vi "jModule - Initialize.vi"(4 "Wait on Module Timeout, ms (5000)":u32=5000, 6 "Wait on Module(s) (\"\": none)":string, 8 "error in (no error)":errorcluster, 9 "jMsgRxList":refnum<class "jMsg.lvclass">[](array[class]), 10 "jMsgTxList":refnum<class "jMsg.lvclass">[](array[class]), 11 "jModule Template_SubPanel UI (Right)":refnum<class "Module_SP_GameLeaderboard.lvclass">) -> (0 "error out":errorcluster, 3 "jModule Template_SubPanel UI (Right)":refnum<class "Module_SP_GameLeaderboard.lvclass">)   [LabVIEW 2019, in "Module_SP_GameLeaderboard.lvclass"]
doc: "This VI is used to intialize the jModule object. \n\nThis includes:\n* Creating the jRouter for the module (the queue for receiving the jMsgs)\n -- Max Queue Size intput limits the number of jMsgs that can back up\n* Adding this module to the subscription list of each message that this module expects to receive (<b>jMsgRxList</b> array)\n* Ensuring that the messages that this module will send (<b>jMsgTxList</b> array) have subscription lists created.\n* Initializing the Timeout for receiving messages to -1\n* Setting up the module to handle Batch jMsg sends\n* Adding the Module Name to the jModuleMasterTable\n* Waiting until every Module listed in the <b>Wait on Module(s)</b> has been added to the jModuleMasterTable\n* Sending out jMsg_Sys_JAMAModuleOnline\n\nNote that ALL modules are automatically registered to:\n* send JAMAException jMsgs\n* receive Shutdown jMsgsJSMA Module Template - SubPanels 0.2.0.9\nRob Humfeld - Jet Engineering\nCopyright (c) 2019, Jet Engineering"
uses:
  Module_SP_GameLeaderboard.lvclass
  C:/Program Files/National Instruments/LabVIEW 2019/user.lib/Jet Engineering/JSMA/Libraries/jModule Class/jModule.lvclass
  <userlib>/Jet Engineering/JSMA/Libraries/jMsg Class/jMsg.lvclass
  <userlib>/Jet Engineering/JSMA Signal Abstraction Layer (SAL)/CORE/jModule_SAL Class/jModule_SAL_ClientRxMsg STYP.ctl
  <userlib>/Jet Engineering/JSMA Signal Abstraction Layer (SAL)/CORE/jMsgs_CORE/jMsg_SAL_TagServiceDefinition/jMsg_SAL_TagServiceDefinition.lvclass
  <userlib>/Jet Engineering/JSMA Signal Abstraction Layer (SAL)/CORE/jMsgs_CORE/jMsg_SAL_TagDataPacket/jMsg_SAL_TagDataPacket.lvclass
  <userlib>/Jet Engineering/JSMA Signal Abstraction Layer (SAL)/CORE/jMsgs_CORE/jMsg_SAL_TagServiceAvailable/jMsg_SAL_TagServiceAvailable.lvclass
  <userlib>/Jet Engineering/JSMA Signal Abstraction Layer (SAL)/CORE/jModule_SAL Class/jModule_SAL_ClientTxMsg STYP.ctl
  <userlib>/Jet Engineering/JSMA Signal Abstraction Layer (SAL)/CORE/jMsgs_CORE/jMsg_SAL_TagServicePoll/jMsg_SAL_TagServicePoll.lvclass
  <userlib>/Jet Engineering/JSMA Signal Abstraction Layer (SAL)/CORE/jMsgs_CORE/jMsg_SAL_TagServiceRequest/jMsg_SAL_TagServiceRequest.lvclass
  <userlib>/Jet Engineering/JSMA/Libraries/jModule Class/jModule.lvclass/jModule.ctl
  <userlib>/Jet Engineering/JSMA/Libraries/jMsg Class/jMsg.lvclass/jMsg.ctl
  <userlib>/Jet Engineering/JSMA/Libraries/jSubscription Class/jSubscription.lvclass/jSubscription.ctl
  <userlib>/Jet Engineering/JSMA/Libraries/jRouter Class/jRouter.lvclass/jRouter.ctl
  <userlib>/Jet Engineering/JSMA/Libraries/jMsg_CORE/jMsg_JSMA_SubscriptionChange/jMsg_JSMA_SubscriptionChange.lvclass/jMsg_JSMA_SubscriptionChange.ctl
  <userlib>/Jet Engineering/JSMA/Libraries/jMsg Class/jMsg Get-Create Subscription List.vi
  <userlib>/Jet Engineering/JSMA/Libraries/jMsg Class/Read Name.vi
  <userlib>/Jet Engineering/JSMA/Libraries/jMasterTable_Message/jMasterTable_Message - Add jMsg.vi
  <userlib>/Jet Engineering/JSMA/Libraries/jMsg_CORE/jMsg_JSMA_SubscriptionChange/(create) jMsg_JSMA_SubscriptionChange.vi
  <userlib>/Jet Engineering/JSMA/Libraries/jModule Class/jModule - SimpleTx.vi
  <userlib>/Jet Engineering/JSMA/Libraries/jSubscription Class/(create) jSubscription.vi
  <userlib>/Jet Engineering/JSMA/Libraries/jSubscription_Background/(create) jSubscription_Background.vi
  <userlib>/Jet Engineering/JSMA/Libraries/jSubscription_Critical/(create) jSubscription_Critical.vi
  <userlib>/Jet Engineering/JSMA/Libraries/jMasterTable_Subscription/jMasterTable_Subscription - Add Subscription.vi
  <userlib>/Jet Engineering/JSMA/Libraries/jMasterTable_Subscription/jMasterTable_Subscription - Get-Create Queue.vi
  <userlib>/Jet Engineering/JSMA/Libraries/Shared/JSMA_GetClassName.vi
  <userlib>/Jet Engineering/JSMA/Libraries/jMasterTable_Message/jMasterTable_Message - Get-Create Queue.vi
  <userlib>/Jet Engineering/JSMA/Libraries/jMsg Class/(create) jMsg.vi
  <userlib>/Jet Engineering/JSMA/Libraries/jMasterTable_Subscription/jMasterTable_Subscription - Remove Module.vi
  <userlib>/Jet Engineering/JSMA/Libraries/jMsg Class/Write Source.vi
  <userlib>/Jet Engineering/JSMA/Libraries/jMasterTable_Subscription/jMasterTable_Subscription - Get Queue Type.vi
  <userlib>/Jet Engineering/JSMA/Libraries/jRouter Class/Read Module RxQueue.vi
  <userlib>/Jet Engineering/JSMA/Libraries/jSubscription Class/Get Module Name.vi
  <userlib>/Jet Engineering/JSMA/Libraries/jSubscription Class/Read jRouter.vi
  <userlib>/Jet Engineering/JSMA/Libraries/jRouter Class/Read Module Name.vi
  <userlib>/Jet Engineering/JSMA/Libraries/jMsg_CORE/jMsg_JSMA_SubscriptionChange/jMsg_JSMA_SubscriptionChange.lvclass
  C:/Program Files/National Instruments/LabVIEW 2019/user.lib/Jet Engineering/JSMA/Libraries/jMsg Class/jMsg.lvclass
  <vilib>/Utility/LVClass/Get LV Class Path.vi
  <userlib>/Jet Engineering/JSMA/Libraries/jModule Class/jModule - Prepare Addressed.vi
  <userlib>/Jet Engineering/JSMA/Libraries/jSubscription Class/jSubscription.lvclass
  <userlib>/Jet Engineering/JSMA/Libraries/jSubscription_Background/jSubscription_Background.lvclass
  <userlib>/Jet Engineering/JSMA/Libraries/jSubscription_Critical/jSubscription_Critical.lvclass
  <userlib>/Jet Engineering/JSMA GUISubPanel CORE/jModule_GUISubPanel.lvclass
  <userlib>/Jet Engineering/JSMA Signal Abstraction Layer (SAL)/CORE/jModule_SAL Class/jModule_SAL_ServerRxMsg STYP.ctl
  <userlib>/JET Engineering/JSMA Signal Abstraction Layer (SAL)/CORE/jModule_SAL Class/jModule_SAL.lvclass
  <userlib>/Jet Engineering/JSMA Signal Abstraction Layer (SAL)/CORE/jModule_SAL Class/jModule_SAL_ServerTxMsg STYP.ctl
  <userlib>/Jet Engineering/JSMA/Libraries/jModule Class/jModule.lvclass
  <userlib>/Jet Engineering/JSMA Signal Abstraction Layer (SAL)/CORE/jMsgs_CORE/jMsg_SAL_SignalUpdate/jMsg_SAL_SignalUpdate.lvclass
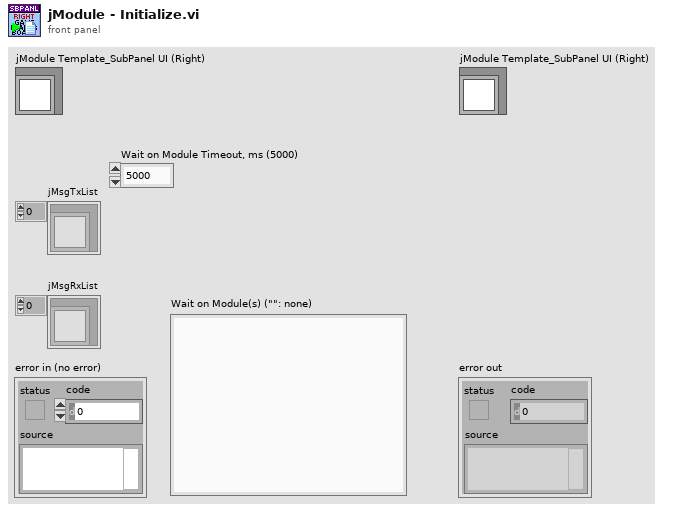
[diagram p1: front panel]
types:
  T1 = typedef "JSMA SAL CORE.lvlib/jModule_SAL.lvclass/jModule_SAL_ServerTxMsg STYP.ctl" = cluster{"jMsg_SAL_TagServiceDefinition":refnum<class "jMsg_SAL_TagServiceDefinition.lvclass">, "jMsg_SAL_TagDataPacket":refnum<class "jMsg_SAL_TagDataPacket.lvclass">, "jMsg_SAL_TagServiceAvailable":refnum<class "jMsg_SAL_TagServiceAvailable.lvclass">}
  T2 = typedef "JSMA SAL CORE.lvlib/jModule_SAL.lvclass/jModule_SAL_ServerRxMsg STYP.ctl" = cluster{"jMsg_SAL_TagServiceRequest":refnum<class "jMsg_SAL_TagServiceRequest.lvclass">, "jMsg_SAL_TagServicePoll":refnum<class "jMsg_SAL_TagServicePoll.lvclass">, "jMsg_SAL_SignalUpdate":refnum<class "jMsg_SAL_SignalUpdate.lvclass">}
  T3 = typedef "JSMA SAL CORE.lvlib/jModule_SAL.lvclass/jModule_SAL_ClientRxMsg STYP.ctl" = cluster{"jMsg_SAL_TagServiceDefinition":refnum<class "jMsg_SAL_TagServiceDefinition.lvclass">, "jMsg_SAL_TagDataPacket":refnum<class "jMsg_SAL_TagDataPacket.lvclass">, "jMsg_SAL_TagServiceAvailable":refnum<class "jMsg_SAL_TagServiceAvailable.lvclass">}
  T4 = typedef "JSMA SAL CORE.lvlib/jModule_SAL.lvclass/jModule_SAL_ClientTxMsg STYP.ctl" = cluster{"jMsg_SAL_TagServicePoll":refnum<class "jMsg_SAL_TagServicePoll.lvclass">, "jMsg_SAL_TagServiceRequest":refnum<class "jMsg_SAL_TagServiceRequest.lvclass">}
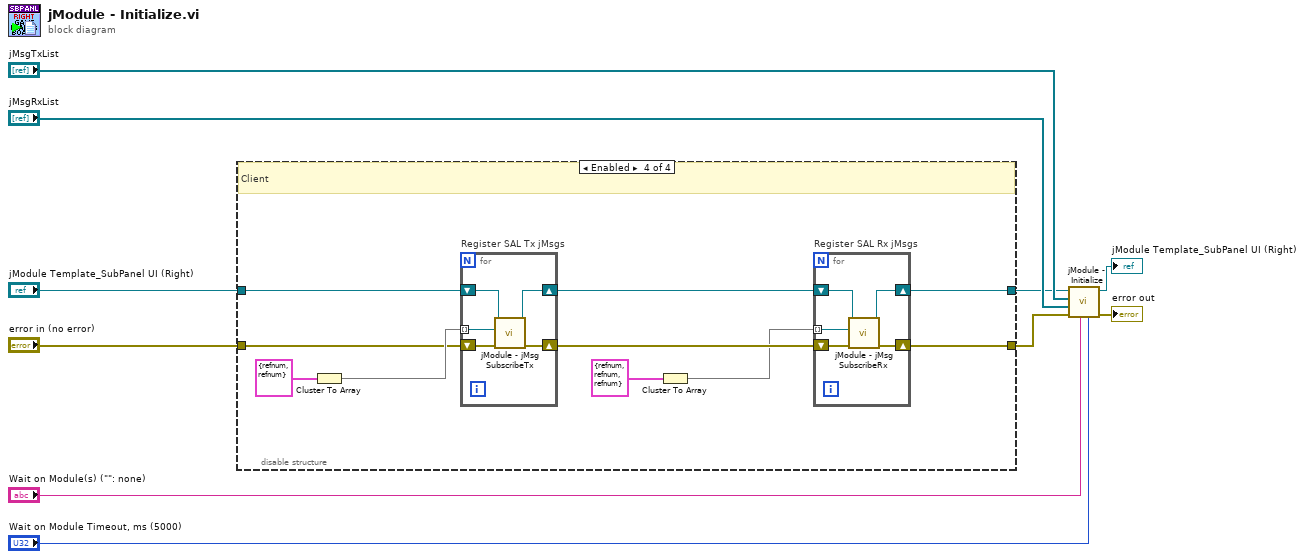
[diagram p0: block diagram]
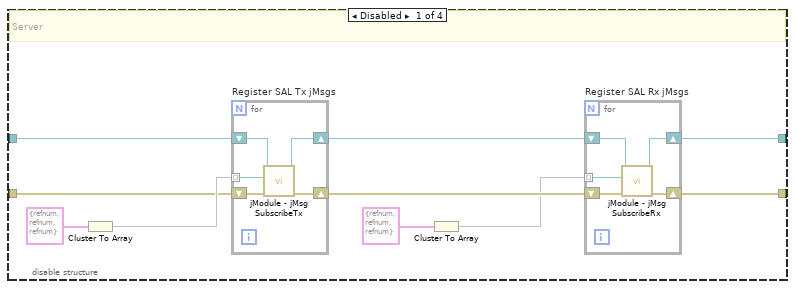
[diagram p2: hidden frame]
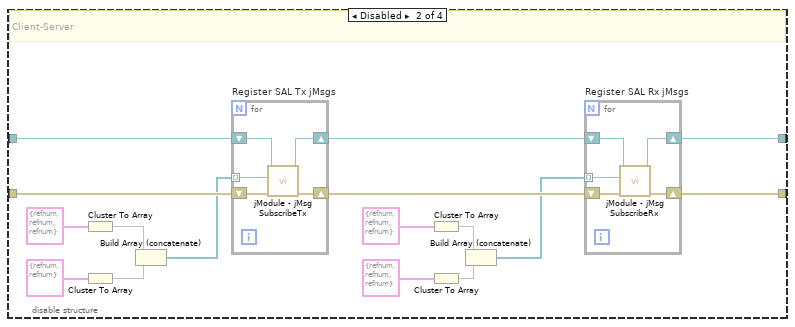
[diagram p3: hidden frame]
diagram:
  n1 = disable-structure shown="Enabled" {
    disable-tunnel: "jModule Template_SubPanel UI (Right)" -> [w15 w42 w58 w62]
    disable-tunnel: [w20 w46 w58 w68] -> w2
    disable-tunnel: "error in (no error)" -> [w14 w41 w57 w61]
    disable-tunnel: [w19 w45 w57 w67] -> w1
    frame Disabled {
      # "Server"
      n2 = Cluster To Array(cluster=T1 {"jMsg_SAL_TagServiceDefinition"=refnum, "jMsg_SAL_TagDataPacket"=refnum, "jMsg_SAL_TagServiceAvailable"=refnum} ("TxMsg")) -> (array=w18:refnum<class "jMsg.lvclass">[])
      n3 = for "Register SAL Tx jMsgs" {
        shift-right: [w29] -> w17
        shift-left: w15 -> [w30]
        tunnel: w18 -> [w28] mode=indexing
        shift-right: [w26] -> w16
        shift-left: w14 -> [w27]
        n4 = call <userlib>:"jModule - jMsg SubscribeTx.vi"("error in (no error)"=w27, "jMsg"=w28, "jModule"=w30) -> ("error out"=w26:errorcluster, "jModule"=w29:refnum<class "Module_SP_GameLeaderboard.lvclass">)  [unwired: 6 in, 1 out]
      }
      n5 = Cluster To Array(cluster=T2 {"jMsg_SAL_TagServiceRequest"=refnum, "jMsg_SAL_TagServicePoll"=refnum, "jMsg_SAL_SignalUpdate"=refnum} ("RxMsg")) -> (array=w13:refnum<class "jMsg.lvclass">[])
      n6 = for "Register SAL Rx jMsgs" {
        shift-right: [w24] -> w20
        shift-left: w17 -> [w25]
        tunnel: w13 -> [w23] mode=indexing
        shift-right: [w21] -> w19
        shift-left: w16 -> [w22]
        n7 = call <userlib>:"jModule - jMsg SubscribeRx.vi"("error in (no error)"=w22, "jMsg"=w23, "jModule"=w25) -> ("error out"=w21:errorcluster, "jModule"=w24:refnum<class "Module_SP_GameLeaderboard.lvclass">)  [unwired: 6 in, 1 out]
      }
    }
    frame Disabled {
      # "Client-Server"
      n8 = Cluster To Array(cluster=T1 {"jMsg_SAL_TagServiceDefinition"=refnum, "jMsg_SAL_TagDataPacket"=refnum, "jMsg_SAL_TagServiceAvailable"=refnum} ("TxMsg")) -> (array=w35:refnum<class "jMsg.lvclass">[])
      n9 = Cluster To Array(cluster=T4 {"jMsg_SAL_TagServicePoll"=refnum, "jMsg_SAL_TagServiceRequest"=refnum} ("TxMsg")) -> (array=w36:refnum<class "jMsg.lvclass">[])
      n10 = Build Array (concatenate)(w35, w36) -> (w34:refnum<class "jMsg.lvclass">[])
      n11 = for "Register SAL Tx jMsgs" {
        shift-right: [w55] -> w44
        shift-left: w42 -> [w56]
        tunnel: w34 -> [w53] mode=indexing
        shift-right: [w52] -> w43
        shift-left: w41 -> [w54]
        n12 = call <userlib>:"jModule - jMsg SubscribeTx.vi"("error in (no error)"=w54, "jMsg"=w53, "jModule"=w56) -> ("error out"=w52:errorcluster, "jModule"=w55:refnum<class "Module_SP_GameLeaderboard.lvclass">)  [unwired: 6 in, 1 out]
      }
      n13 = Cluster To Array(cluster=T2 {"jMsg_SAL_TagServiceRequest"=refnum, "jMsg_SAL_TagServicePoll"=refnum, "jMsg_SAL_SignalUpdate"=refnum} ("RxMsg")) -> (array=w32:refnum<class "jMsg.lvclass">[])
      n14 = Cluster To Array(cluster=T3 {"jMsg_SAL_TagServiceDefinition"=refnum, "jMsg_SAL_TagDataPacket"=refnum, "jMsg_SAL_TagServiceAvailable"=refnum} ("RxMsg")) -> (array=w33:refnum<class "jMsg.lvclass">[])
      n15 = Build Array (concatenate)(w32, w33) -> (w31:refnum<class "jMsg.lvclass">[])
      n16 = for "Register SAL Rx jMsgs" {
        shift-right: [w50] -> w46
        shift-left: w44 -> [w51]
        tunnel: w31 -> [w47] mode=indexing
        shift-right: [w48] -> w45
        shift-left: w43 -> [w49]
        n17 = call <userlib>:"jModule - jMsg SubscribeRx.vi"("error in (no error)"=w49, "jMsg"=w47, "jModule"=w51) -> ("error out"=w48:errorcluster, "jModule"=w50:refnum<class "Module_SP_GameLeaderboard.lvclass">)  [unwired: 6 in, 1 out]
      }
    }
    frame Disabled {
      # "jModule_SAL Parent Class"
    }
    frame Enabled {
      # "Client"
      n18 = Cluster To Array(cluster=T4 {"jMsg_SAL_TagServicePoll"=refnum, "jMsg_SAL_TagServiceRequest"=refnum} ("TxMsg")) -> (array=w66:refnum<class "jMsg.lvclass">[])
      n19 = for "Register SAL Tx jMsgs" {
        shift-right: [w77] -> w64
        shift-left: w62 -> [w78]
        tunnel: w66 -> [w75] mode=indexing
        shift-right: [w74] -> w63
        shift-left: w61 -> [w76]
        n20 = call <userlib>:"jModule - jMsg SubscribeTx.vi"("error in (no error)"=w76, "jMsg"=w75, "jModule"=w78) -> ("error out"=w74:errorcluster, "jModule"=w77:refnum<class "Module_SP_GameLeaderboard.lvclass">)  [unwired: 6 in, 1 out]
      }
      n21 = Cluster To Array(cluster=T3 {"jMsg_SAL_TagServiceDefinition"=refnum, "jMsg_SAL_TagDataPacket"=refnum, "jMsg_SAL_TagServiceAvailable"=refnum} ("RxMsg")) -> (array=w59:refnum<class "jMsg.lvclass">[])
      n22 = for "Register SAL Rx jMsgs" {
        shift-right: [w72] -> w68
        shift-left: w64 -> [w73]
        tunnel: w59 -> [w69] mode=indexing
        shift-right: [w70] -> w67
        shift-left: w63 -> [w71]
        n23 = call <userlib>:"jModule - jMsg SubscribeRx.vi"("error in (no error)"=w71, "jMsg"=w69, "jModule"=w73) -> ("error out"=w70:errorcluster, "jModule"=w72:refnum<class "Module_SP_GameLeaderboard.lvclass">)  [unwired: 6 in, 1 out]
      }
    }
  }
  n24 = call-parent "jModule - Initialize.vi"("Wait on Module Timeout, ms (5000)"="Wait on Module Timeout, ms (5000)", "Wait on Module(s) (\"\": none)"="Wait on Module(s) (\"\": none)", "error in (no error)"=w1, "jMsgRxList"="jMsgRxList", "jMsgTxList"="jMsgTxList", "jModule_GUISubPanel"=w2) -> ("error out"=→"error out":errorcluster, "jModule_GUISubPanel"=→"jModule Template_SubPanel UI (Right)":refnum<class "Module_SP_GameLeaderboard.lvclass">)  [unwired: 4 in]
